vi "To Pretty String (String).vi"(0 "Variant in":variant, 5 "indent":i32, 11 "error in (no error)":errorcluster) -> (4 "String":string, 15 "error out":errorcluster)   [LabVIEW 2017, in "Advanced Variant Tools.lvlib"]
doc: "Flattens the given JSON data to a string."
uses:
  Advanced Variant Tools.lvlib
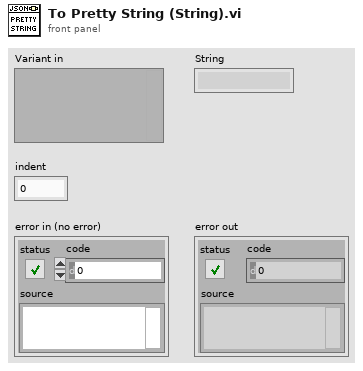
[diagram p1: front panel]
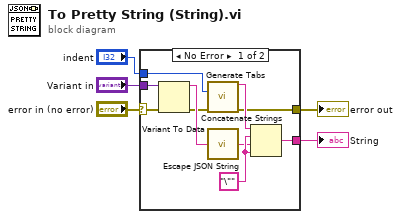
[diagram p0: block diagram]
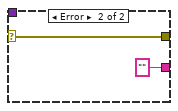
[diagram p2: hidden frame]
diagram:
  n1 = case shown="No Error" "error in (no error)" {
    selector: "error in (no error)" -> [w7 w16]
    tunnel: "Variant in" -> [w8 _]
    tunnel: [w14 ""] -> w4
    tunnel: [w10 w16] -> w3
    tunnel: "indent" -> [w12 _]
    frame No Error {
      w15 = "\"" ("string")
      n2 = Variant To Data(error in=w7, Variant=w8) -> (data=w9:string, error out=w6:errorcluster)  [unwired: 1 in]
      n3 = call "Generate Tabs.vi"("indent"=w12, "error in (no error)"=w6) -> ("Tabs"=w11:string, "error out"=w10:errorcluster)  [unwired: 12 in]
      n4 = call "Escape JSON String.vi"("value"=w9) -> ("escaped string"=w13:string)  [unwired: 14 in]
      n5 = Concatenate Strings(w11, w15, w13, w15) -> (w14:string)
    }
    frame Error {
    }
  }
  "String" <- w4
  "error out" <- w3
